vi "Launcher.vi"   [LabVIEW 2019]
uses:
  GameLogic/GameLogic/GameLogic.lvclass
  C:/Program Files (x86)/National Instruments/LabVIEW 2019/vi.lib/ActorFramework/Actor/Actor.lvclass
  <vilib>/ActorFramework/Actor/Actor.lvclass
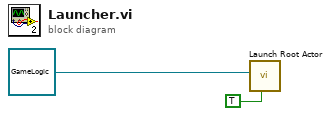
[diagram p0: block diagram]
diagram:
  n1 = call <vilib>:"Launch Root Actor.vi"("Open Actor Core front panel? (F)"=TRUE, "Actor"=refnum<class "GameLogic.lvclass"> refnum ("GameLogic.lvlib:GameLogic.lvclass")) -> ()  [unwired: 8 in, 2 out]
